vi "Trans Convertor.vi"(11 "operation":T2 items=["Direct", "Conjugated & Transposed", "Transposed"]) -> (3 "trans":T1=111 items=["CblasNoTrans"=111, "CblasTrans"=112, "CblasConjTrans "=113])   [LabVIEW 2017, in "NI_AALBLAS.lvlib"]
uses:
  <vilib>/Analysis/NI_AALBLAS.lvlib
  <vilib>/Analysis/BLAS.llb/LV_Transpose.ctl
  <vilib>/Analysis/BLAS.llb/Operation_Transpose.ctl
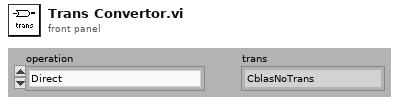
[diagram p1: front panel]
types:
  T1 = typedef "NI_AALBLAS.lvlib/Operation_Transpose.ctl" = i32
  T2 = typedef "NI_AALBLAS.lvlib/LV_Transpose.ctl" = i32
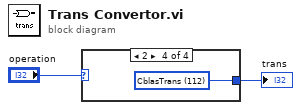
[diagram p0: block diagram]
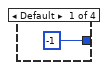
[diagram p2: hidden frame]
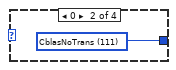
[diagram p3: hidden frame]
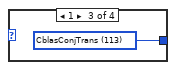
[diagram p4: hidden frame]
diagram:
  n1 = case shown="2" "operation" {
    tunnel: [-1 w4 w5 w6] -> w1
    frame Default {
    }
    frame 0 {
      w4 = T1 111 items=["CblasNoTrans"=111, "CblasTrans"=112, "CblasConjTrans "=113] ("trans 2")
    }
    frame 1 {
      w5 = T1 113 items=["CblasNoTrans"=111, "CblasTrans"=112, "CblasConjTrans "=113] ("trans 2")
    }
    frame 2 {
      w6 = T1 112 items=["CblasNoTrans"=111, "CblasTrans"=112, "CblasConjTrans "=113] ("trans 2")
    }
  }
  "trans" <- w1
